vi "EMI_project_v4.vi"() -> ()   [LabVIEW 2020]
uses:
  <vilib>/Instr/_visa.llb/VISA Flush IO Buffer Mask.ctl
  <vilib>/Analysis/baseanly.llb/Mean (DBL).vi
  <vilib>/Instr/_visa.llb/VISA Configure Serial Port (Instr).vi
  <vilib>/Analysis/NI_AALBase.lvlib
panel:
  out "Take Average CH02":bool
  out "Take Average CH01":bool
  out "Voltage Peak CH02":dynamicdata(graph)
  out "Voltage Peak CH01":dynamicdata(graph)
  in  "stop 2":bool
  out "Voltage Thresould CH 2":dbl
  in  "Noise Thresould 2":dbl
  in  "Take Average CH 2":bool
  out "Voltage Thresould CH 01":dbl
  in  "Noise Thresould":dbl
  in  "Take Average CH 01":bool
  out "Fader 02 level":dbl
  out "Fader 01 level":dbl
  out "Gain Knob 02 level":dbl
  out "Gain knob 01 level":dbl
  out "manual mode led":bool
  out "Sound Balance Mode":bool
  in  "Gain Knob 02":dbl(knob) scale=0.0..270.0
  in  "Gain Knob 01":dbl(knob) scale=0.0..270.0
  in  "Fader 02 Slider":dbl(slide) scale=0.0..10.0
  in  "Fader 01 Slider":dbl(slide) scale=0.0..10.0
  out "Fader 02 Max":dbl
  out "Fader 01 Max":dbl
  in  "Calibrate":bool
  in  "stop":bool
  in  "VISA Resource":refnum<visa-resource-name>
  in  "?":bool
  in  "Gain 02":bool
  in  "?":bool
  in  "Gain 01":bool
  in  "?":bool
  in  "Fader 02":bool
  in  "?":bool
  in  "Fader 01":bool
  # "Automation System For Analog Audio Mixers"
  # "Calibration \nMode"
  # "Manual Mode"
  # "Sound Balance Mode"
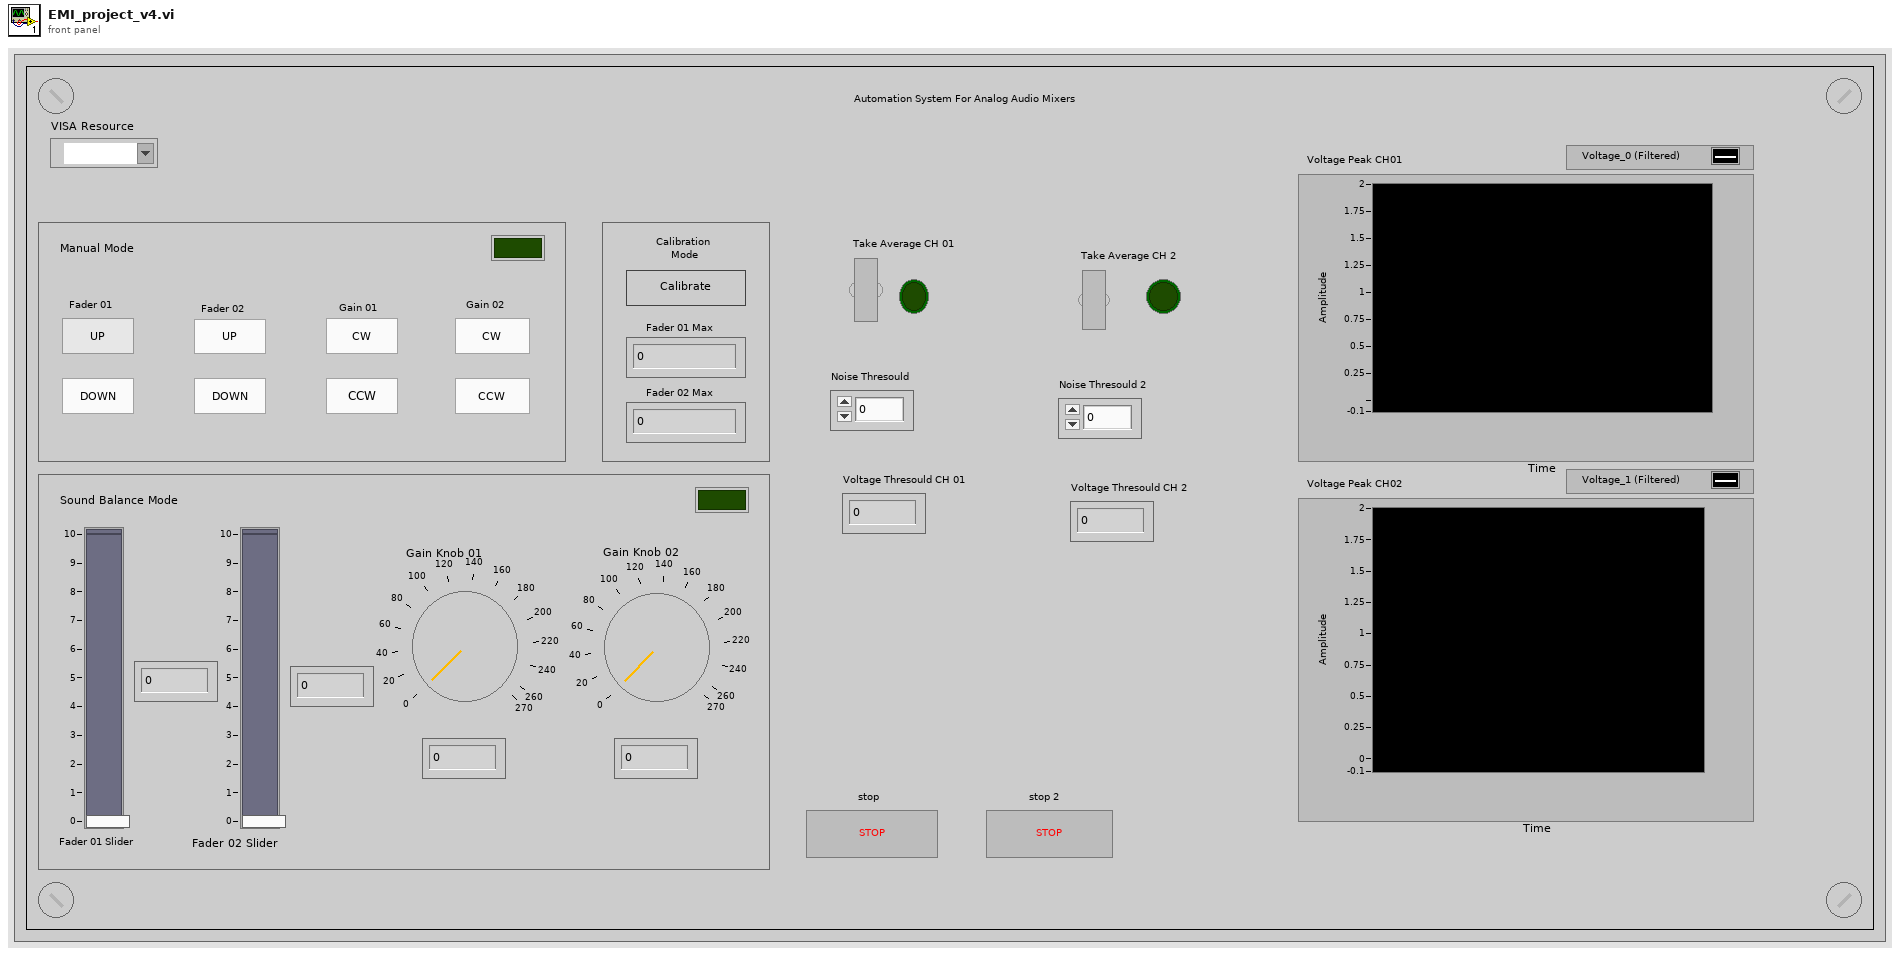
[diagram p1: front panel]
types:
  T1 = typedef "VISA Flush IO Buffer Mask.ctl" = u16
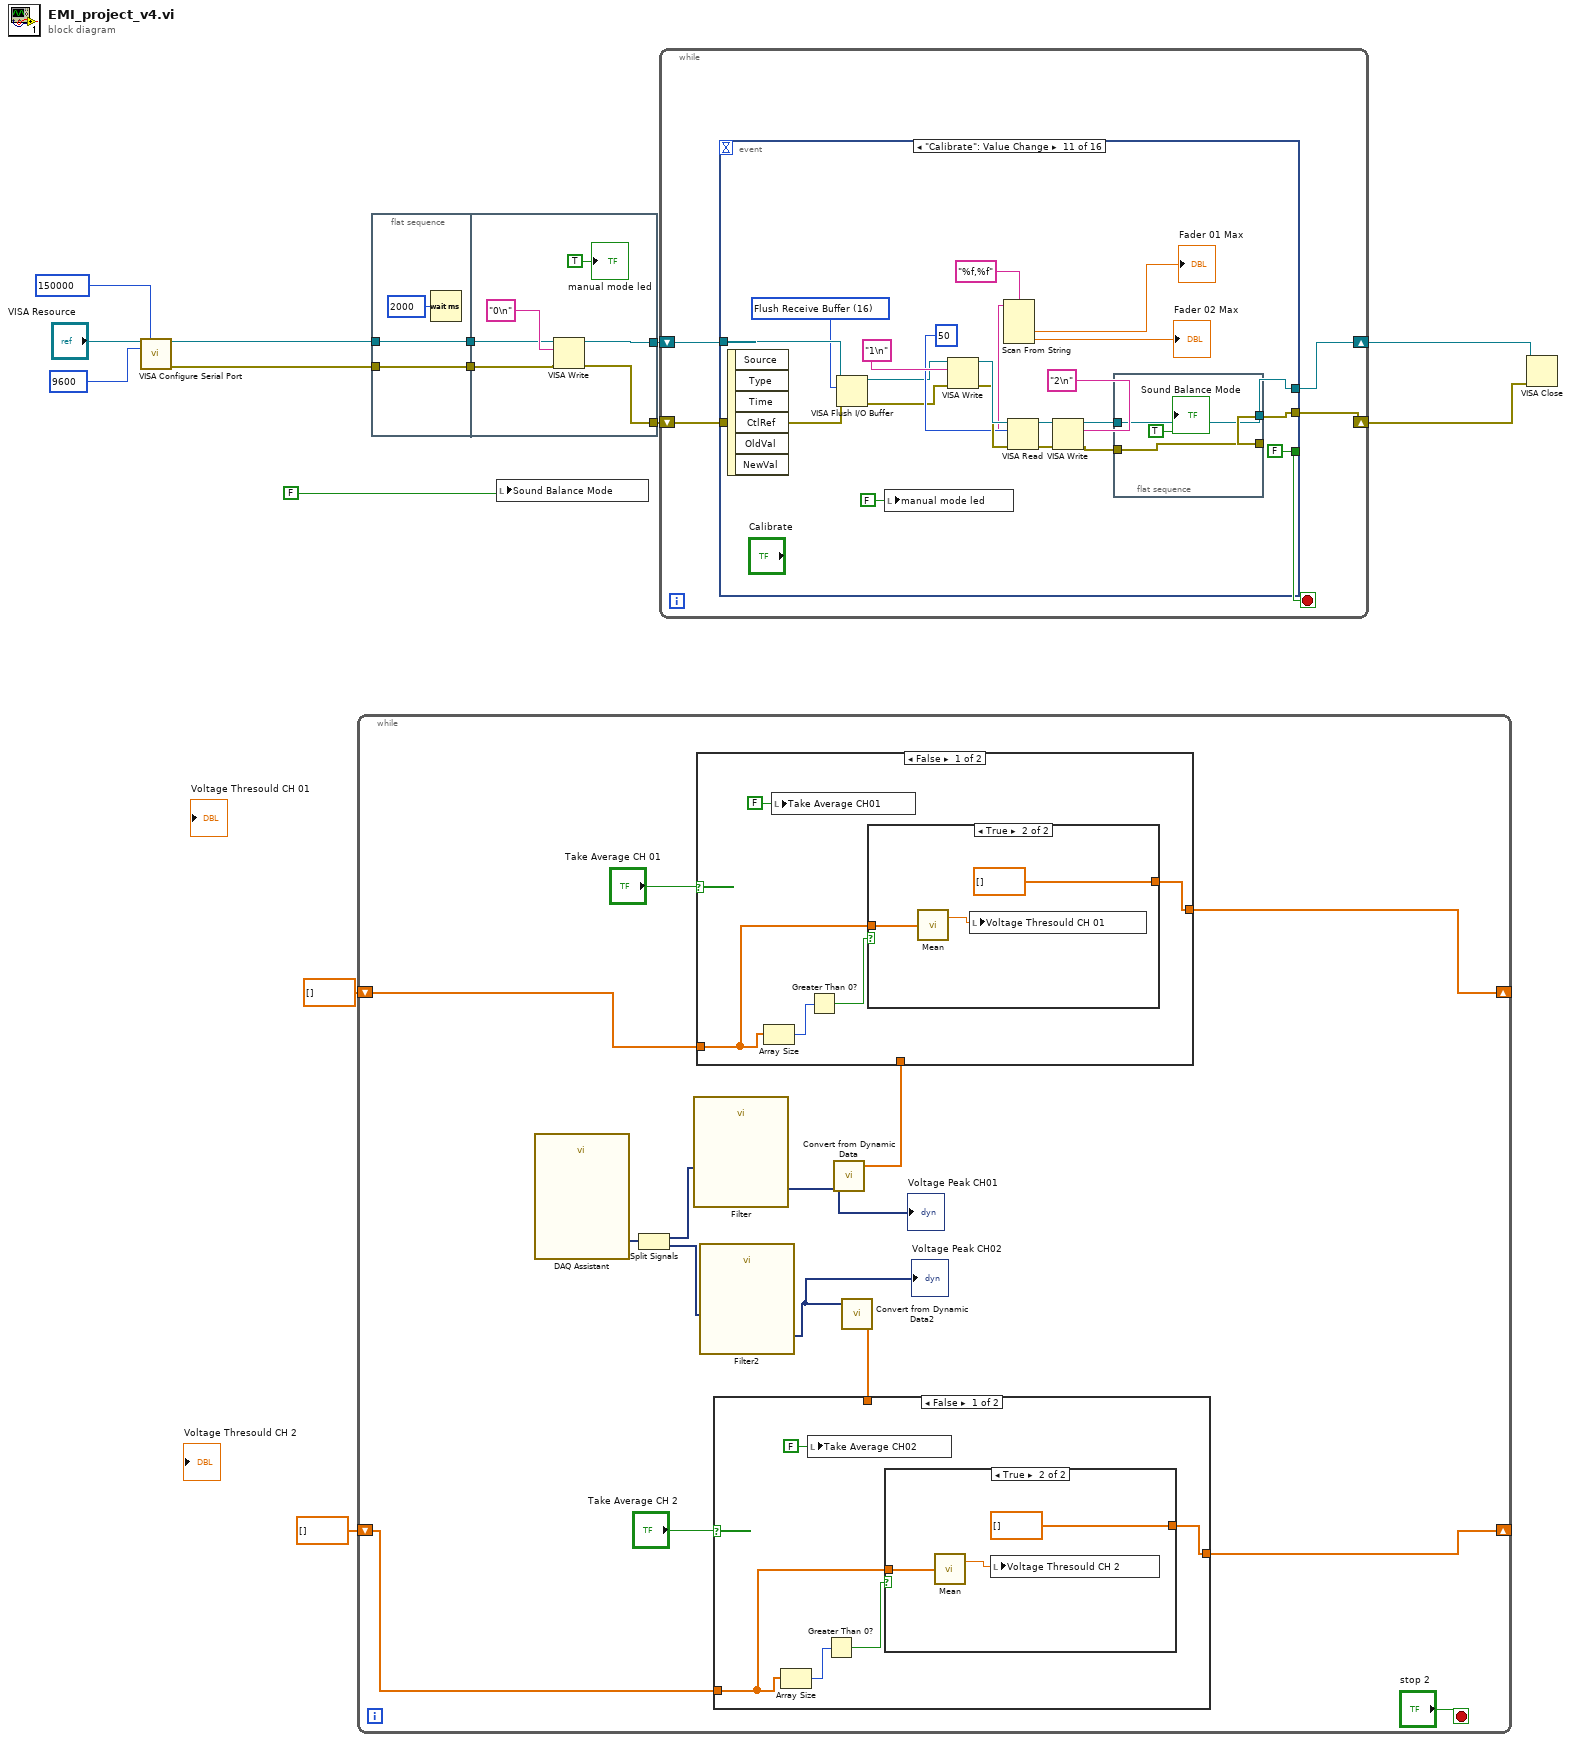
[diagram p0: block diagram]
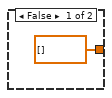
[diagram p2: hidden frame]
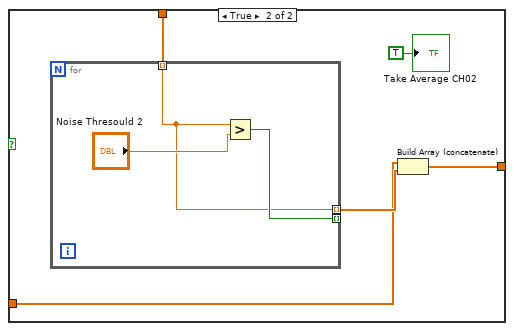
[diagram p3: hidden frame]
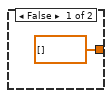
[diagram p4: hidden frame]
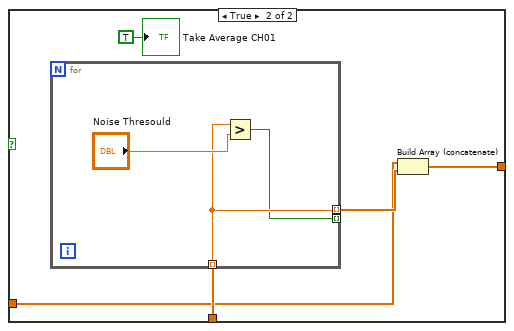
[diagram p5: hidden frame]
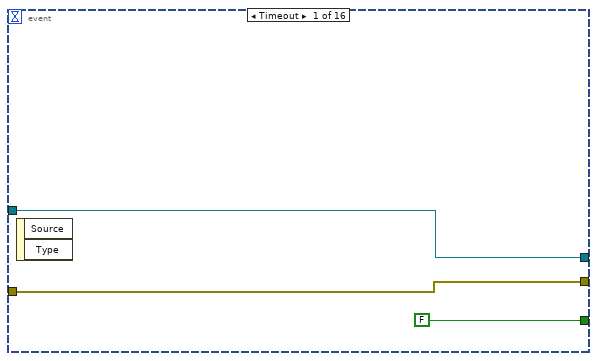
[diagram p6: hidden frame]
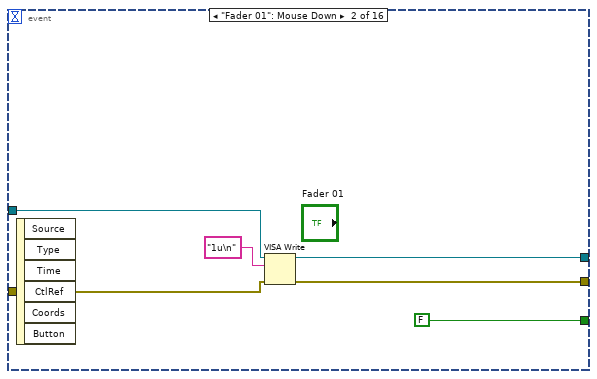
[diagram p7: hidden frame]
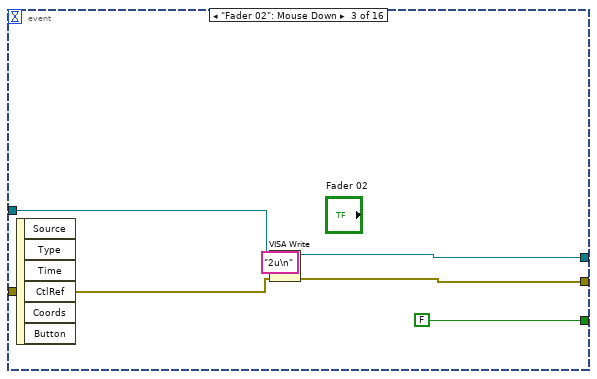
[diagram p8: hidden frame]
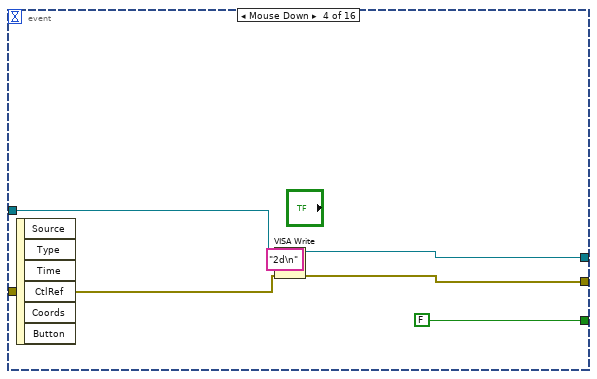
[diagram p9: hidden frame]
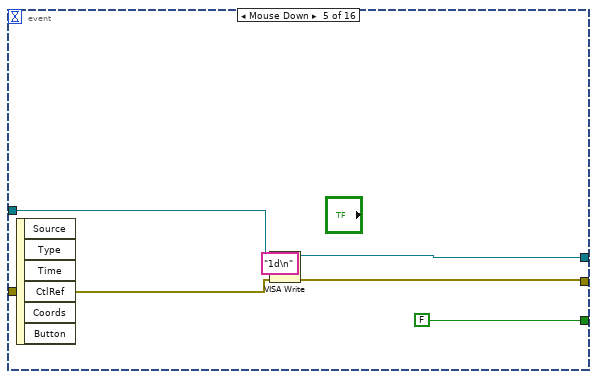
[diagram p10: hidden frame]
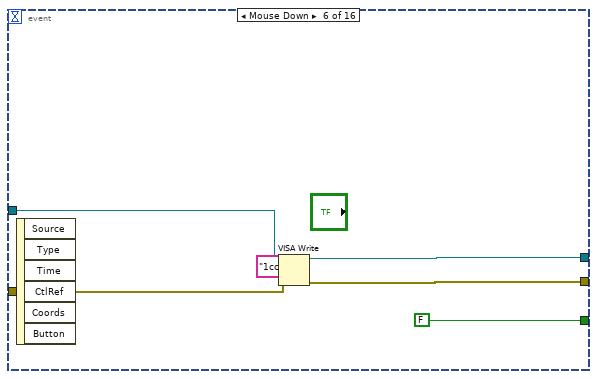
[diagram p11: hidden frame]
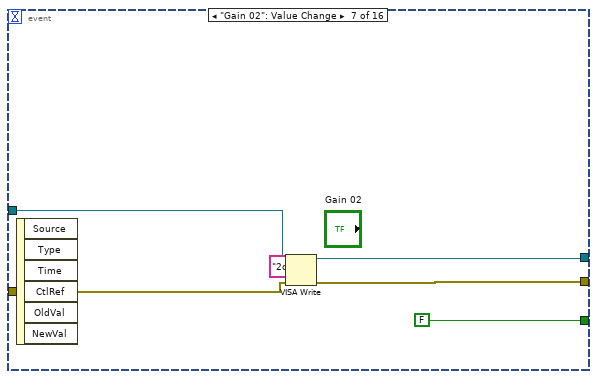
[diagram p12: hidden frame]
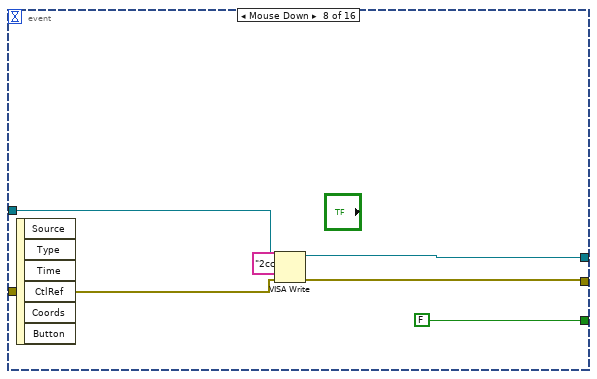
[diagram p13: hidden frame]
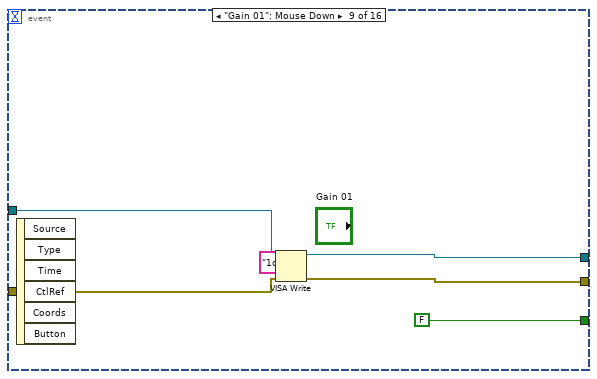
[diagram p14: hidden frame]
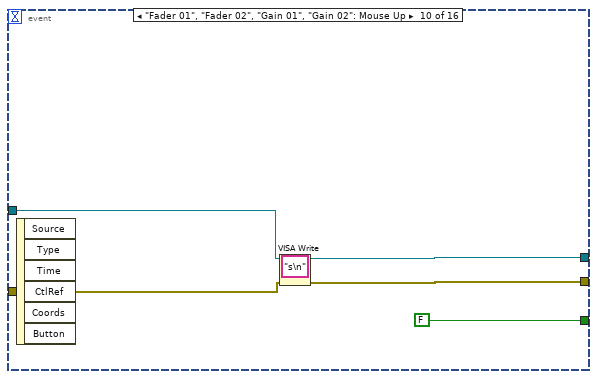
[diagram p15: hidden frame]
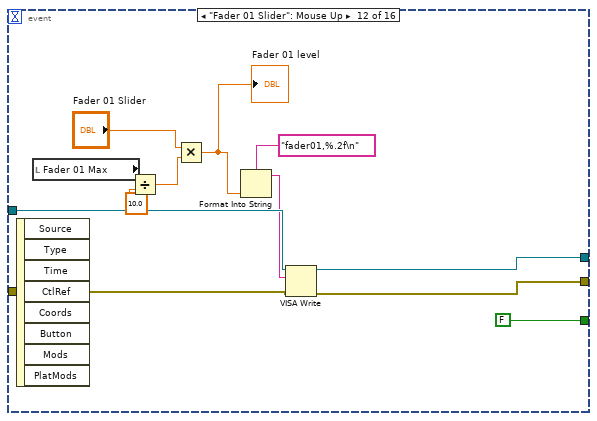
[diagram p16: hidden frame]
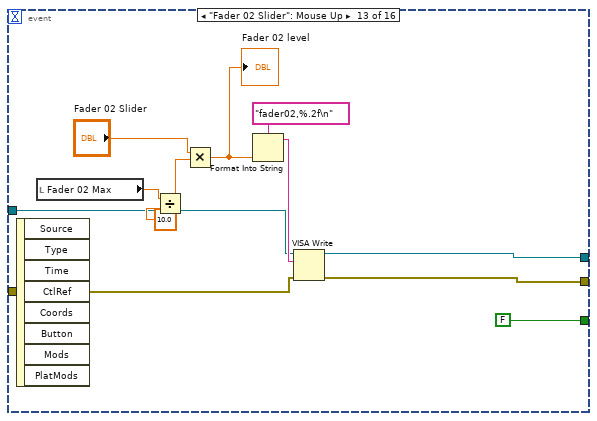
[diagram p17: hidden frame]
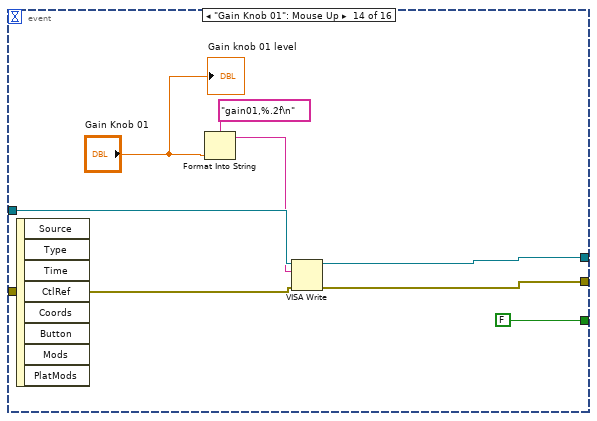
[diagram p18: hidden frame]
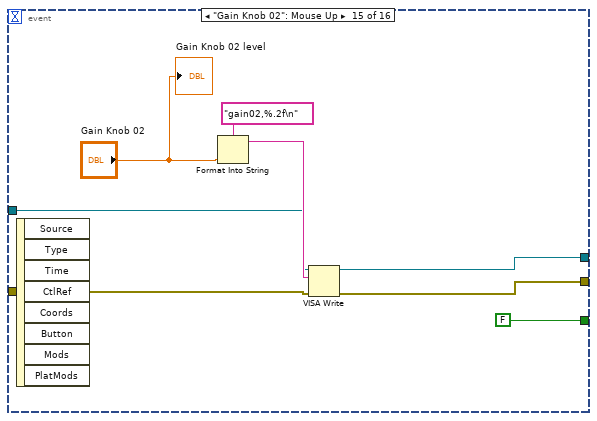
[diagram p19: hidden frame]
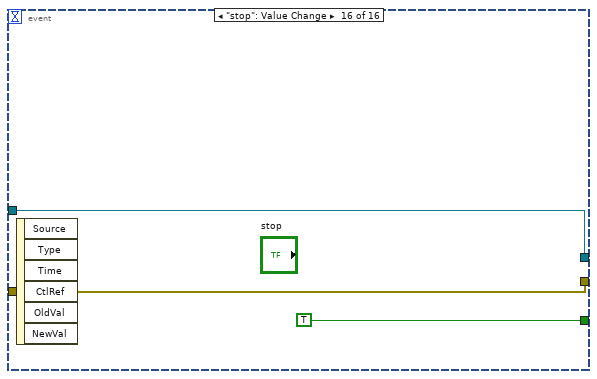
[diagram p20: hidden frame]
diagram:
  n1 = call-poly "VISA Configure Serial Port"("VISA resource name"="VISA Resource", "timeout (10sec)"=u32 150000, "baud rate (9600)"=u32 9600) -> ("VISA resource name out"=w8:refnum<visa-resource-name>, "error out"=w7:errorcluster)  [unwired: 11 in]
  n2 = while {
    shift-right: [w22] -> _
    shift-left: dbl[] [] -> [w23]
    shift-right: [w20] -> _
    shift-left: dbl[] [] -> [w18]
    stop <- "stop 2" stop-if-true
    n3 = call "DAQ Assistant"() -> ("data"=w27:dynamicdata)  [unwired: 16 in, 3 out]
    n4 = Split Signals(w27) -> (w26:dynamicdata, w25:dynamicdata)  [unwired: 2 in]
    n5 = call "Filter"("Signal"=w26) -> ("Filtered Signal"=w16:dynamicdata)  [unwired: 9 in, 1 out]
    "Voltage Peak CH01" <- w16
    n6 = call "Filter2"("Signal"=w25) -> ("Filtered Signal"=w15:dynamicdata)  [unwired: 9 in, 1 out]
    "Voltage Peak CH02" <- w15
    n7 = call "Convert from Dynamic Data"("Dynamic Data Type"=w16) -> ("Array"=w24:dbl[])  [unwired: 3 in]
    n8 = case shown="False" "Take Average CH 01" {
      tunnel: w24 -> [_ w59]
      tunnel: w23 -> [w48 w56]
      tunnel: [w47 w57] -> w22
      frame False {
        n9 = Array Size(array=w48) -> (size(s)=w50:i32)
        n10 = local write "Take Average CH01"(FALSE ("Take Average CH01")) -> ()
        n11 = Greater Than 0?(x=w50) -> (x > 0?=w49:bool)
        n12 = case shown="True" w49 {
          tunnel: w48 -> [_ w54]
          tunnel: [dbl[] [] dbl[] []] -> w47
          frame False {
          }
          frame True {
            n13 = call-poly <vilib>:"Mean.vi"("X"=w54) -> ("mean"=w53:dbl)  [unwired: 1 out]
            n14 = local write "Voltage Thresould CH 01"(w53) -> ()
          }
        }
      }
      frame True {
        n15 = for {
          tunnel: w59 -> [w61] mode=indexing
          tunnel: [w61] -> w58 mode=indexing if=w60
          tunnel: [w60] -> _ mode=indexing
          n16 = Greater?(x=w61, y="Noise Thresould") -> (0:w60:bool)
        }
        n17 = Build Array (concatenate)(w56, w58) -> (w57:dbl[])
        "Take Average CH01" <- TRUE ("Take Average CH01")
      }
    }
    n18 = call "Convert from Dynamic Data2"("Dynamic Data Type"=w15) -> ("Array"=w19:dbl[])  [unwired: 3 in]
    n19 = case shown="False" "Take Average CH 2" {
      tunnel: w18 -> [w31 w41]
      tunnel: [w30 w40] -> w20
      tunnel: w19 -> [_ w39]
      frame False {
        n20 = Array Size(array=w31) -> (size(s)=w33:i32)
        n21 = local write "Take Average CH02"(FALSE ("Take Average CH02")) -> ()
        n22 = Greater Than 0?(x=w33) -> (x > 0?=w32:bool)
        n23 = case shown="True" w32 {
          tunnel: w31 -> [_ w37]
          tunnel: [dbl[] [] dbl[] []] -> w30
          frame False {
          }
          frame True {
            n24 = call-poly <vilib>:"Mean.vi"("X"=w37) -> ("mean"=w36:dbl)  [unwired: 1 out]
            n25 = local write "Voltage Thresould CH 2"(w36) -> ()
          }
        }
      }
      frame True {
        n26 = for {
          tunnel: [w43] -> w42 mode=indexing if=w44
          tunnel: [w44] -> _ mode=indexing
          tunnel: w39 -> [w43] mode=indexing
          n27 = Greater?(x=w43, y="Noise Thresould 2") -> (0:w44:bool)
        }
        n28 = Build Array (concatenate)(w41, w42) -> (w40:dbl[])
        "Take Average CH02" <- TRUE ("Take Average CH02")
      }
    }
  }
  n29 = flat-sequence {
    tunnel: w7 -> [w64]
    tunnel: w8 -> [w65]
    tunnel: [w65] -> w6
    tunnel: [w64] -> w5
    tunnel: [w70] -> w12
    tunnel: [w69] -> w11
    tunnel: w6 -> [w68]
    tunnel: w5 -> [w67]
    frame #0 {
      n30 = Wait (ms)(milliseconds to wait=u32 2000) -> ()  [unwired: 1 out]
    }
    frame #1 {
      n31 = VISA Write(VISA resource name=w68, write buffer="0\n", error in (no error)=w67) -> (VISA resource name out=w70:refnum<visa-resource-name>, error out=w69:errorcluster)  [unwired: 1 out]
      "manual mode led" <- TRUE
    }
  }
  n32 = local write "Sound Balance Mode"(FALSE) -> ()
  n33 = while {
    shift-right: [w74] -> w10
    shift-left: w12 -> [w76]
    shift-right: [w73] -> w9
    shift-left: w11 -> [w75]
    stop <- w72 stop-if-true
    n34 = event shown="[10] \"Calibrate\": Value Change" {
      selector: _ -> [_ _ _ _ _ _ _ _ _ _ _ _ _ _ _ _]
      dyn-events: _ -> [_ _ _ _ _ _ _ _ _ _ _ _ _ _ _ _]
      timeout: _ -> [_ _ _ _ _ _ _ _ _ _ _ _ _ _ _ _]
      tunnel: w76 -> [w79 w85 w89 w95 w103 w106 w113 w119 w125 w131 w147 w165 w176 w189 w196 w200]
      tunnel: w75 -> [w78 w84 w88 w94 w102 w107 w112 w118 w124 w130 w146 w164 w175 w188 w195 w199]
      tunnel: [w79 w82 w91 w97 w100 w109 w115 w121 w127 w133 w138 w161 w173 w186 w193 w200] -> w74
      tunnel: [w78 w81 w90 w96 w101 w108 w114 w120 w126 w132 w135 w163 w174 w187 w194 w199] -> w73
      tunnel: [FALSE FALSE FALSE FALSE FALSE FALSE FALSE FALSE FALSE FALSE FALSE FALSE FALSE FALSE FALSE TRUE] -> w72
      event Timeout {
        n35 = event-data() -> ()  [unwired: 1 in, 2 out]
      }
      event "Fader 01": Mouse Down {
        n36 = event-data() -> ()  [unwired: 1 in, 6 out]
        n37 = VISA Write(VISA resource name=w85, write buffer="1u\n", error in (no error)=w84) -> (VISA resource name out=w82:refnum<visa-resource-name>, error out=w81:errorcluster)  [unwired: 1 out]
      }
      event "Fader 02": Mouse Down {
        n38 = event-data() -> ()  [unwired: 1 in, 6 out]
        n39 = VISA Write(VISA resource name=w89, write buffer="2u\n", error in (no error)=w88) -> (VISA resource name out=w91:refnum<visa-resource-name>, error out=w90:errorcluster)  [unwired: 1 out]
      }
      event Mouse Down {
        n40 = event-data() -> ()  [unwired: 1 in, 6 out]
        n41 = VISA Write(VISA resource name=w95, write buffer="2d\n", error in (no error)=w94) -> (VISA resource name out=w97:refnum<visa-resource-name>, error out=w96:errorcluster)  [unwired: 1 out]
      }
      event Mouse Down {
        n42 = event-data() -> ()  [unwired: 1 in, 6 out]
        n43 = VISA Write(VISA resource name=w103, write buffer="1d\n", error in (no error)=w102) -> (VISA resource name out=w100:refnum<visa-resource-name>, error out=w101:errorcluster)  [unwired: 1 out]
      }
      event Mouse Down {
        n44 = event-data() -> ()  [unwired: 1 in, 6 out]
        n45 = VISA Write(VISA resource name=w106, write buffer="1ccw\n", error in (no error)=w107) -> (VISA resource name out=w109:refnum<visa-resource-name>, error out=w108:errorcluster)  [unwired: 1 out]
      }
      event "Gain 02": Value Change {
        n46 = event-data() -> ()  [unwired: 1 in, 6 out]
        n47 = VISA Write(VISA resource name=w113, write buffer="2cw\n", error in (no error)=w112) -> (VISA resource name out=w115:refnum<visa-resource-name>, error out=w114:errorcluster)  [unwired: 1 out]
      }
      event Mouse Down {
        n48 = event-data() -> ()  [unwired: 1 in, 6 out]
        n49 = VISA Write(VISA resource name=w119, write buffer="2ccw\n", error in (no error)=w118) -> (VISA resource name out=w121:refnum<visa-resource-name>, error out=w120:errorcluster)  [unwired: 1 out]
      }
      event "Gain 01": Mouse Down {
        n50 = event-data() -> ()  [unwired: 1 in, 6 out]
        n51 = VISA Write(VISA resource name=w125, write buffer="1cw\n", error in (no error)=w124) -> (VISA resource name out=w127:refnum<visa-resource-name>, error out=w126:errorcluster)  [unwired: 1 out]
      }
      event "Fader 01", "Fader 02", "Gain 01", "Gain 02": Mouse Up {
        n52 = event-data() -> ()  [unwired: 1 in, 6 out]
        n53 = VISA Write(VISA resource name=w131, write buffer="s\n", error in (no error)=w130) -> (VISA resource name out=w133:refnum<visa-resource-name>, error out=w132:errorcluster)  [unwired: 1 out]
      }
      event "Calibrate": Value Change {
        w143 = T1 16 items=["Flush Receive Buffer"=16, "Write Transmit Buffer to Device"=32, "Flush Receive Buffer (No I/O)"=64, "Flush Transmit Buffer"=128] ("Mask")
        n54 = event-data() -> ()  [unwired: 1 in, 6 out]
        n55 = VISA Flush I/O Buffer(VISA resource name=w147, mask (16)=w143, error in (no error)=w146) -> (VISA resource name out=w145:refnum<visa-resource-name>, error out=w144:errorcluster)
        n56 = local write "manual mode led"(FALSE ("manual mode led")) -> ()
        n57 = VISA Write(VISA resource name=w145, write buffer="1\n", error in (no error)=w144) -> (VISA resource name out=w154:refnum<visa-resource-name>, error out=w153:errorcluster)  [unwired: 1 out]
        n58 = VISA Read(VISA resource name=w154, byte count=u32 50, error in (no error)=w153) -> (VISA resource name out=w142:refnum<visa-resource-name>, read buffer=w151:string, error out=w141:errorcluster)  [unwired: 1 out]
        n59 = Scan From String(format string="%f,%f", input string=w151) -> (output 1=→"Fader 01 Max":dbl, output 2=→"Fader 02 Max":dbl)  [unwired: 4 in, 3 out]
        n60 = VISA Write(VISA resource name=w142, write buffer="2\n", error in (no error)=w141) -> (VISA resource name out=w137:refnum<visa-resource-name>, error out=w136:errorcluster)  [unwired: 1 out]
        n61 = flat-sequence {
          tunnel: [w157] -> w138
          tunnel: w137 -> [w157]
          tunnel: w136 -> [w156]
          tunnel: [w156] -> w135
          frame #0 {
            "Sound Balance Mode" <- TRUE
          }
        }
      }
      event "Fader 01 Slider": Mouse Up {
        n62 = event-data() -> ()  [unwired: 1 in, 8 out]
        n63 = local read "Fader 01 Max"() -> (w169:dbl)
        n64 = Divide(x=w169, y=10.0) -> (x/y=w166:dbl)
        n65 = Multiply(x="Fader 01 Slider", y=w166) -> (x*y=w159:dbl)
        "Fader 01 level" <- w159
        n66 = Format Into String(format string="fader01,%.2f\n", w159) -> (resulting string=w160:string)  [unwired: 2 in, 1 out]
        n67 = VISA Write(VISA resource name=w165, write buffer=w160, error in (no error)=w164) -> (VISA resource name out=w161:refnum<visa-resource-name>, error out=w163:errorcluster)  [unwired: 1 out]
      }
      event "Fader 02 Slider": Mouse Up {
        n68 = event-data() -> ()  [unwired: 1 in, 8 out]
        n69 = local read "Fader 02 Max"() -> (w182:dbl)
        n70 = Divide(x=w182, y=10.0) -> (x/y=w179:dbl)
        n71 = Multiply(x="Fader 02 Slider", y=w179) -> (x*y=w171:dbl)
        "Fader 02 level" <- w171
        n72 = Format Into String(format string="fader02,%.2f\n", w171) -> (resulting string=w177:string)  [unwired: 2 in, 1 out]
        n73 = VISA Write(VISA resource name=w176, write buffer=w177, error in (no error)=w175) -> (VISA resource name out=w173:refnum<visa-resource-name>, error out=w174:errorcluster)  [unwired: 1 out]
      }
      event "Gain Knob 01": Mouse Up {
        n74 = event-data() -> ()  [unwired: 1 in, 8 out]
        n75 = Format Into String(format string="gain01,%.2f\n", "Gain Knob 01") -> (resulting string=w185:string)  [unwired: 2 in, 1 out]
        n76 = VISA Write(VISA resource name=w189, write buffer=w185, error in (no error)=w188) -> (VISA resource name out=w186:refnum<visa-resource-name>, error out=w187:errorcluster)  [unwired: 1 out]
        "Gain knob 01 level" <- "Gain Knob 01"
      }
      event "Gain Knob 02": Mouse Up {
        n77 = event-data() -> ()  [unwired: 1 in, 8 out]
        n78 = Format Into String(format string="gain02,%.2f\n", "Gain Knob 02") -> (resulting string=w197:string)  [unwired: 2 in, 1 out]
        n79 = VISA Write(VISA resource name=w196, write buffer=w197, error in (no error)=w195) -> (VISA resource name out=w193:refnum<visa-resource-name>, error out=w194:errorcluster)  [unwired: 1 out]
        "Gain Knob 02 level" <- "Gain Knob 02"
      }
      event "stop": Value Change {
        n80 = event-data() -> ()  [unwired: 1 in, 6 out]
      }
    }
  }
  n81 = VISA Close(VISA resource name=w10, error in (no error)=w9) -> ()  [unwired: 1 out]
